vi "highTarget.vi"(1 "4":dbl[][](array[numeric]), 2 "3":dbl[][](array[numeric]), 3 "2":dbl[][](array[numeric]), 4 "1":dbl[][](array[numeric])) -> (0 "Highest Y":dbl[][](array[numeric]))   [LabVIEW 2011]
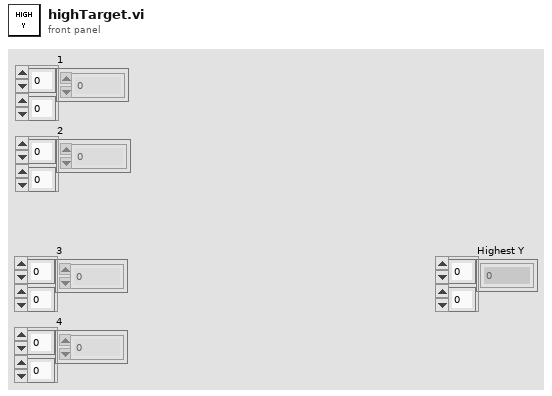
[diagram p1: front panel]
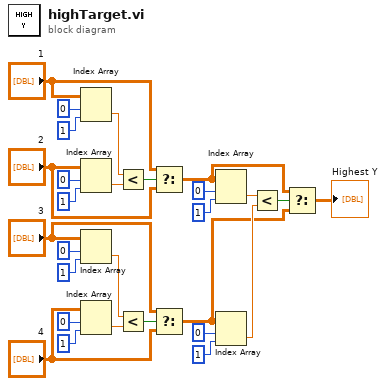
[diagram p0: block diagram]
diagram:
  n1 = Index Array(array="1", index (row)=0 ("disabled index (row)"), index (col)=1 ("disabled index (col)")) -> (element=w14:dbl)
  n2 = Index Array(array="2", index (row)=0 ("disabled index (row)"), index (col)=1 ("disabled index (col)")) -> (element=w15:dbl)
  n3 = Index Array(array="3", index (row)=0 ("disabled index (row)"), index (col)=1 ("disabled index (col)")) -> (element=w27:dbl)
  n4 = Index Array(array="4", index (row)=0 ("disabled index (row)"), index (col)=1 ("disabled index (col)")) -> (element=w26:dbl)
  n5 = Less?(x=w14, y=w15) -> (x < y?=w18:bool)
  n6 = Less?(x=w27, y=w26) -> (x < y?=w23:bool)
  n7 = Select(t="1", s=w18, f="2") -> (s? t:f=w1:dbl[][])
  n8 = Select(t="3", s=w23, f="4") -> (s? t:f=w2:dbl[][])
  n9 = Index Array(array=w1, index (row)=0 ("disabled index (row)"), index (col)=1 ("disabled index (col)")) -> (element=w13:dbl)
  n10 = Index Array(array=w2, index (row)=0 ("disabled index (row)"), index (col)=1 ("disabled index (col)")) -> (element=w12:dbl)
  n11 = Less?(x=w13, y=w12) -> (x < y?=w28:bool)
  n12 = Select(t=w1, s=w28, f=w2) -> (s? t:f=→"Highest Y":dbl[][])
